vi "mWmotor_get_move_Setp_limits.vi"(0 "VISA resource name":refnum<visa-resource-name>, 11 "error in (no error)":errorcluster) -> (3 "Current":bool, 4 "VISA resource name out":refnum<visa-resource-name>, 6 "Move":bool, 8 "Revolutions":dbl, 10 "Positive_L":bool, 14 "error out":errorcluster, 15 "Negetive_L":bool)   [LabVIEW 2019]
panel:
  in  "milliseconds to wait":u32=100
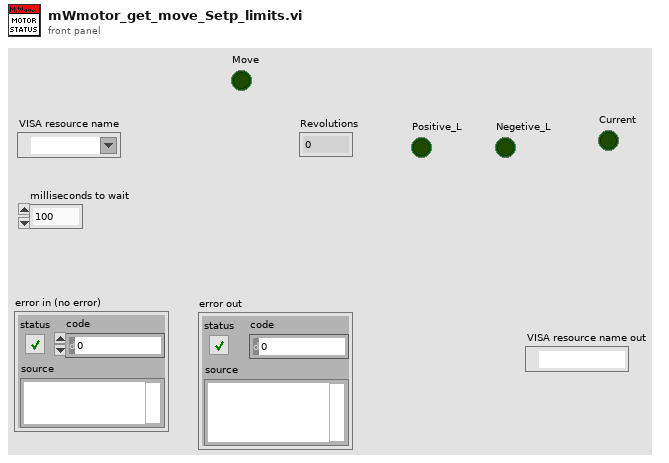
[diagram p1: front panel]
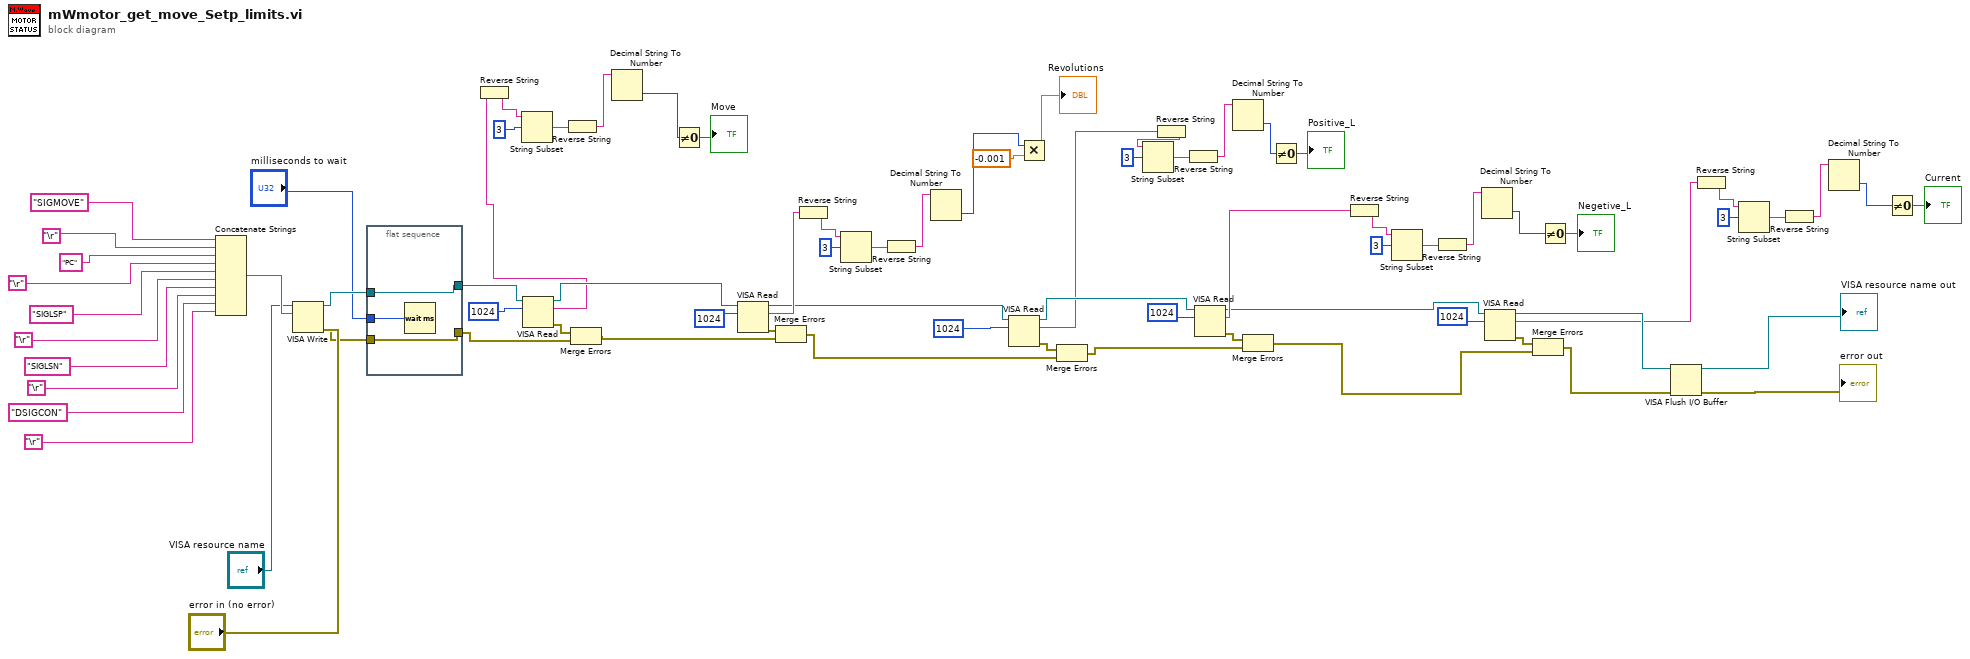
[diagram p0: block diagram]
diagram:
  n1 = Concatenate Strings("SIGMOVE" ("string"), "\r", "PC" ("string"), "\r", "SIGLSP" ("string"), "\r", "SIGLSN" ("string"), "\r", "DSIGCON" ("string"), "\r") -> (w76:string)
  n2 = VISA Write(VISA resource name="VISA resource name", write buffer=w76, error in (no error)="error in (no error)") -> (VISA resource name out=w71:refnum<visa-resource-name>, error out=w72:errorcluster)  [unwired: 1 out]
  n3 = flat-sequence {
    tunnel: [w79] -> w66
    tunnel: w72 -> [w79]
    tunnel: [w78] -> w70
    tunnel: w71 -> [w78]
    tunnel: "milliseconds to wait" -> [w77]
    frame #0 {
      n4 = Wait (ms)(milliseconds to wait=w77) -> ()  [unwired: 1 out]
    }
  }
  n5 = VISA Read(VISA resource name=w70, byte count=u32 1024) -> (VISA resource name out=w55:refnum<visa-resource-name>, read buffer=w20:string, error out=w65:errorcluster)  [unwired: 1 in, 1 out]
  n6 = Reverse String(1:w20) -> (0:w24:string)
  n7 = String Subset(string=w24, offset (0)=3) -> (substring=w23:string)  [unwired: 1 in]
  n8 = Reverse String(1:w23) -> (0:w22:string)
  n9 = Merge Errors(w65, w66) -> (w56:errorcluster)
  n10 = Decimal String To Number(string=w22) -> (number=w21:i32)  [unwired: 2 in, 1 out]
  n11 = Not Equal To 0?(x=w21) -> (x != 0?=→"Move":bool)
  n12 = VISA Read(VISA resource name=w55, byte count=u32 1024) -> (VISA resource name out=w46:refnum<visa-resource-name>, read buffer=w61:string, error out=w62:errorcluster)  [unwired: 1 in, 1 out]
  n13 = Merge Errors(w62, w56) -> (w47:errorcluster)
  n14 = Reverse String(1:w61) -> (0:w59:string)
  n15 = String Subset(string=w59, offset (0)=3) -> (substring=w58:string)  [unwired: 1 in]
  n16 = Reverse String(1:w58) -> (0:w57:string)
  n17 = Decimal String To Number(string=w57) -> (number=w18:i32)  [unwired: 2 in, 1 out]
  n18 = VISA Read(VISA resource name=w46, byte count=u32 1024) -> (VISA resource name out=w40:refnum<visa-resource-name>, read buffer=w35:string, error out=w49:errorcluster)  [unwired: 1 in, 1 out]
  n19 = Multiply(x=w18, y=-0.001) -> (x*y=→"Revolutions":dbl)
  n20 = Merge Errors(w49, w47) -> (w41:errorcluster)
  n21 = Reverse String(1:w35) -> (0:w38:string)
  n22 = String Subset(string=w38, offset (0)=3) -> (substring=w37:string)  [unwired: 1 in]
  n23 = Reverse String(1:w37) -> (0:w36:string)
  n24 = VISA Read(VISA resource name=w40, byte count=u32 1024) -> (VISA resource name out=w4:refnum<visa-resource-name>, read buffer=w29:string, error out=w43:errorcluster)  [unwired: 1 in, 1 out]
  n25 = Decimal String To Number(string=w36) -> (number=w34:i32)  [unwired: 2 in, 1 out]
  n26 = Merge Errors(w43, w41) -> (w5:errorcluster)
  n27 = Not Equal To 0?(x=w34) -> (x != 0?=→"Positive_L":bool)
  n28 = Reverse String(1:w29) -> (0:w32:string)
  n29 = String Subset(string=w32, offset (0)=3) -> (substring=w31:string)  [unwired: 1 in]
  n30 = Reverse String(1:w31) -> (0:w30:string)
  n31 = Decimal String To Number(string=w30) -> (number=w28:i32)  [unwired: 2 in, 1 out]
  n32 = VISA Read(VISA resource name=w4, byte count=u32 1024) -> (VISA resource name out=w3:refnum<visa-resource-name>, read buffer=w1:string, error out=w7:errorcluster)  [unwired: 1 in, 1 out]
  n33 = Merge Errors(w7, w5) -> (w2:errorcluster)
  n34 = Not Equal To 0?(x=w28) -> (x != 0?=→"Negetive_L":bool)
  n35 = VISA Flush I/O Buffer(VISA resource name=w3, error in (no error)=w2) -> (VISA resource name out=→"VISA resource name out":refnum<visa-resource-name>, error out=→"error out":errorcluster)  [unwired: 1 in]
  n36 = Reverse String(1:w1) -> (0:w10:string)
  n37 = String Subset(string=w10, offset (0)=3) -> (substring=w11:string)  [unwired: 1 in]
  n38 = Reverse String(1:w11) -> (0:w12:string)
  n39 = Decimal String To Number(string=w12) -> (number=w13:i32)  [unwired: 2 in, 1 out]
  n40 = Not Equal To 0?(x=w13) -> (x != 0?=→"Current":bool)
